vi "RT_main.vi"() -> ()   [LabVIEW 2013]
uses:
  <vilib>/NI/STM/compatibility/stm_MetaDataElement.ctl
  <vilib>/Platform/TimedLoop/XDataNode/timing_clust.ctl
  <vilib>/Platform/TimedLoop/XDataNode/nitl_modes.ctl
  <vilib>/Platform/TimedLoop/XDataNode/wakeup.ctl
  <vilib>/NI/STM/compatibility/stm_TCP Read Options.ctl
  <vilib>/rvi/interface/common/niFpgaWaitOnOcc.vi
  <vilib>/NI/STM/TCP/Get Connection Reference (TCP).vi
  <vilib>/NI/STM/TCP/Write Meta Data (TCP Ref).vi
  <vilib>/FPGAPlugInAG/cRIO-9101/niLvFpga_Open_cRIO-9101.vi
  <vilib>/rvi/interface/common/dynamic/niFpgaDynamicAddResources.vi
  <vilib>/FPGAPlugInAG/Dynamic/niLvFpga_Reset_Dynamic.vi
  <vilib>/FPGAPlugInAG/Dynamic/niLvFpga_Run_Dynamic.vi
  <vilib>/Utility/error.llb/Error Cluster From Error Code.vi
  <vilib>/rvi/errors/niLvFpgaAdjustHostInterfaceError.vi
  <vilib>/NI/STM/TCP/Read Message (TCP).vi
  <vilib>/NI/STM/TCP/Write Message (TCP).vi
  <vilib>/FPGAPlugInAG/Dynamic/niLvFpga_Close_Dynamic.vi
  <vilib>/Platform/TimedLoop/XDataNode/XDataNode.xnode
  <vilib>/rvi/interface/nirviOpenFPGA/nirviOpenFPGA.xnode
  FPGA Bitfiles/ForceClamp_FPGATarget_FPGAMain_Jp-CpyR53JY.lvbitx
  FPGA_Main.vi
  <vilib>/rvi/interface/nirviMethod/nirviMethod.xnode
  <vilib>/rvi/interface/nirviReadWriteControl/nirviReadWriteControl.xnode
  <vilib>/rvi/interface/nirviCloseFPGA/nirviCloseFPGA.xnode
  <vilib>/rvi/errors/niLvFpgaMergeErrorWithErrorCode.vi
  <vilib>/NI/STM/NI STM.lvlib
  <vilib>/rvi/interface/Simulation/niFpgaSimulationCallBeginRW.vi
  <vilib>/FPGAPlugInAG/Dynamic/niLvFpga_StartFifo_Dynamic.vi
  <vilib>/FPGAPlugInAG/Dynamic/niLvFpga_ReadFifo_Dynamic.vi
  <vilib>/FPGAPlugInAG/Dynamic/niLvFpga_ConfigureFifo_Dynamic.vi
  <vilib>/Platform/TimedLoop/XDataNode/XDNodeRunTimeDep.lvlib
  <vilib>/FPGAPlugInAG/Dynamic/niLvFpga_StopFifo_Dynamic.vi
  <vilib>/FPGAPlugInAG/Dynamic/niLvFpga_WriteFifo_Dynamic.vi
  NiFpgaLv.dll
panel:
  out "Receive Loop Timing":u32
  out "New waveTable":bool
  in  "Repeat mode":bool
  out "Data":fxp<+/-,20,5>[](array[numeric])
  out "Send Loop Timing":u32
  out "Connection OK":bool
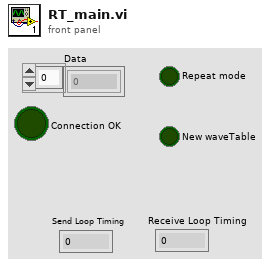
[diagram p1: front panel]
types:
  T1 = typedef "stm_MetaDataElement.ctl" = string
  T2 = typedef "Semaphore RefNum" = refnum<k1>
  T3 = typedef "NI STM.lvlib/TCP Connection Info.ctl" = cluster{"connection ID":refnum<k5>, "Meta data":T4[]}
  T4 = typedef "NI STM.lvlib/MetaDataElement.ctl" = string
  T5 = typedef "XDNodeRunTimeDep.lvlib/timing_clust.ctl" = cluster{"Expected End [f-1]":u64, "Actual End [f-1]":u64, "Finished Late? [f-1]":bool, "Expected End [i-1]":u64, "Actual End [i-1]":u64, "Finished Late? [i-1]":bool, "Expected Start [i]":u64, "Actual Start [i]":u64, "Expected Start [f]":u64, "Actual Start [f]":u64, "Source Name":string, "Structure Name":string, "Period":i64, "Deadline":i64, "Offset":i64, "Start":i64, "Priority":i32, "Timeout":i32, "Mode":T6, "Wakeup Reason":T7, "Error":errorcluster, "Source Type":string, "Secondary Source Type":string, "Global End Time":u64, "Global Start Time":u64, "Frame Duration":u64, "Iteration Duration":u64, "Assigned CPU":i32, "I/O Scan Engine Mode":u32}
  T6 = typedef "XDNodeRunTimeDep.lvlib/nitl_modes.ctl" = enum32{"No Change", "Process missed periods, maintain original phase", "Discard missed periods, maintain original phase", "Process missed periods, ignore original phase", "Discard missed periods, ignore original phase"}
  T7 = typedef "XDNodeRunTimeDep.lvlib/wakeup.ctl" = enum32{"Normal", "Aborted", "Asynchronous wakeup", "Timing source error", "Timed loop error", "Timeout"}
  T8 = typedef "stm_TCP Read Options.ctl" = cluster{"Ignore Timeout Error":bool, "timeout ms (1000)":i32}
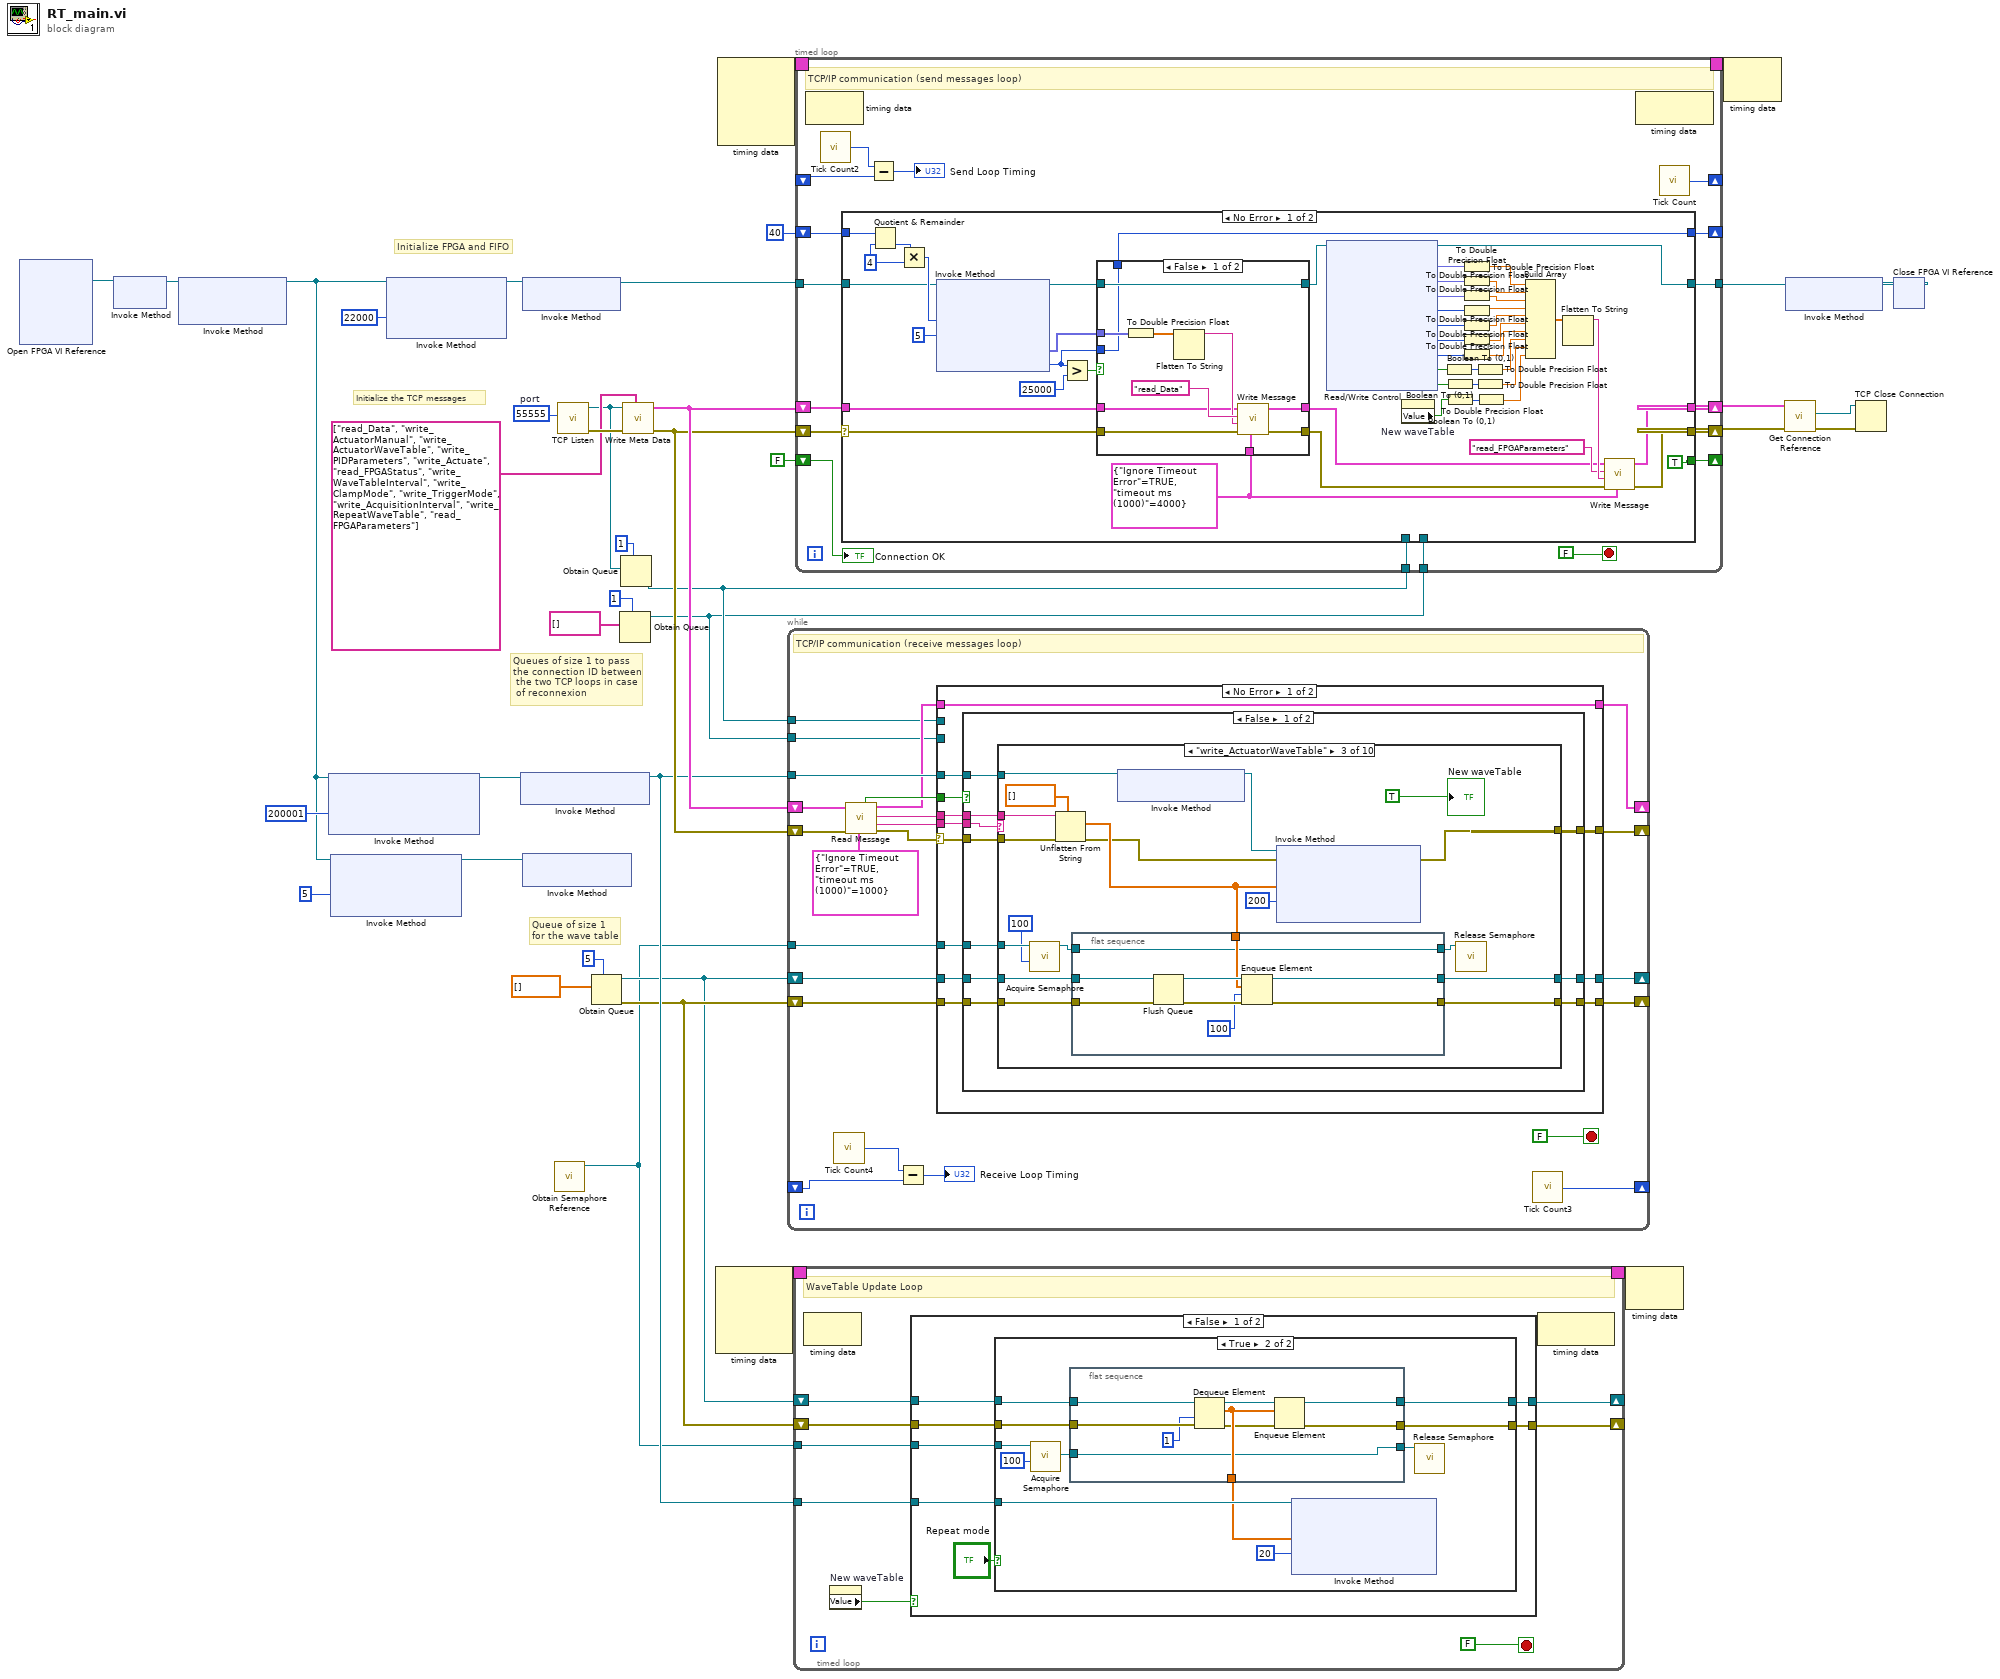
[diagram p0: block diagram]
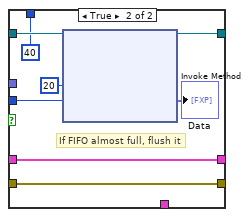
[diagram p2: hidden frame]
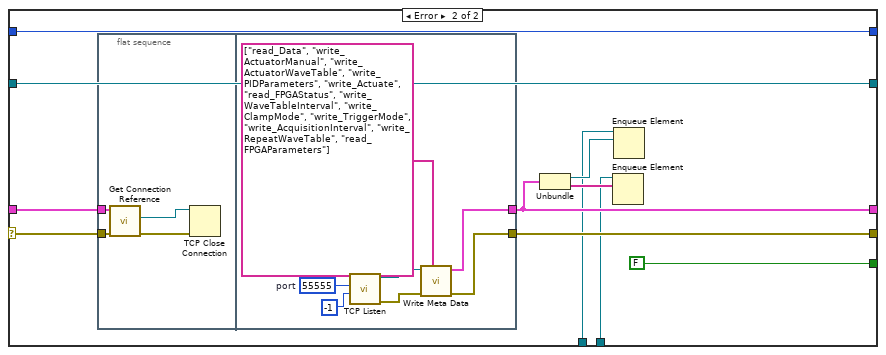
[diagram p3: hidden frame]
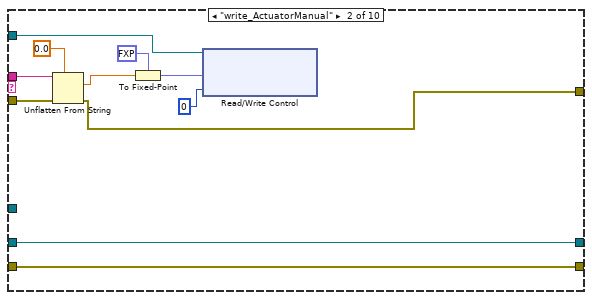
[diagram p5: hidden frame]
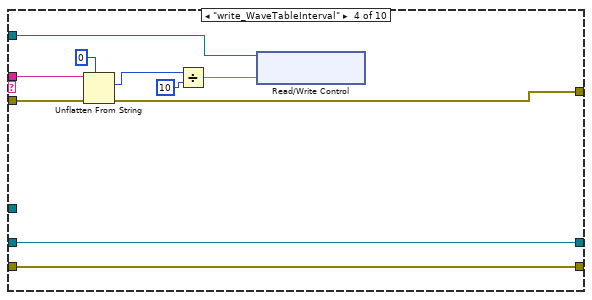
[diagram p6: hidden frame]
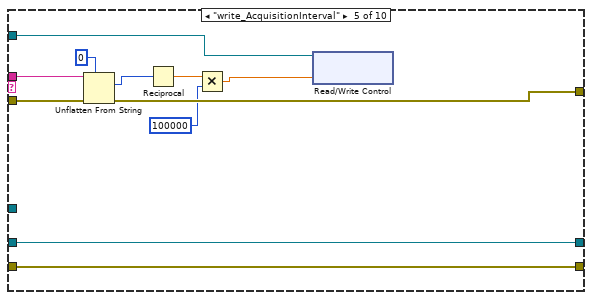
[diagram p7: hidden frame]
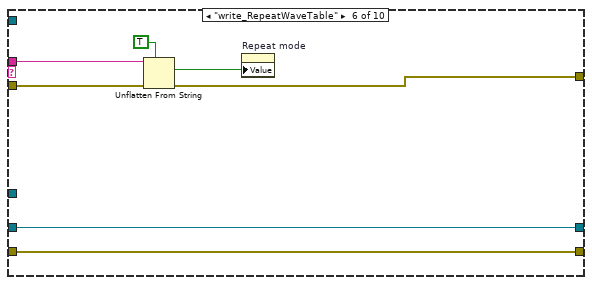
[diagram p8: hidden frame]
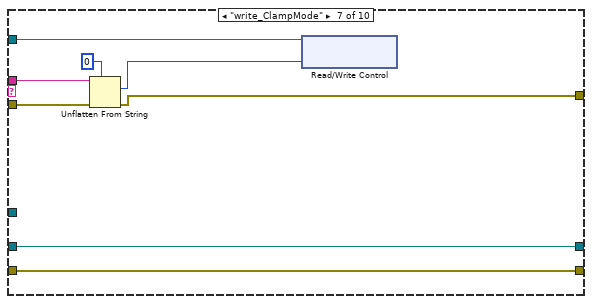
[diagram p9: hidden frame]
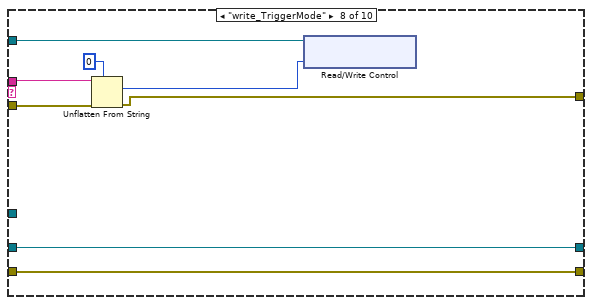
[diagram p10: hidden frame]
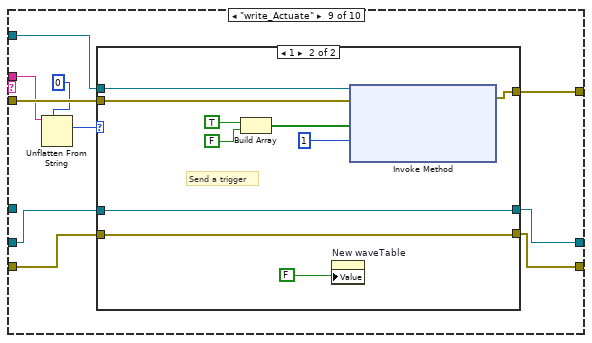
[diagram p11: hidden frame]
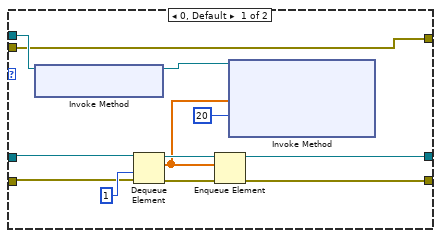
[diagram p12: hidden frame]
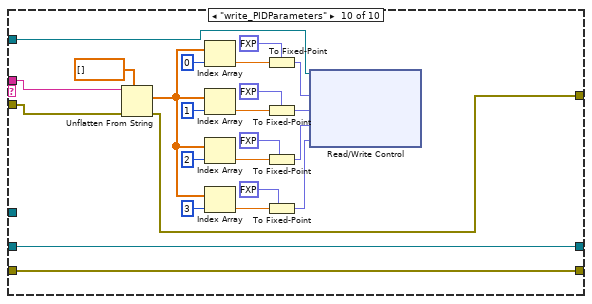
[diagram p13: hidden frame]
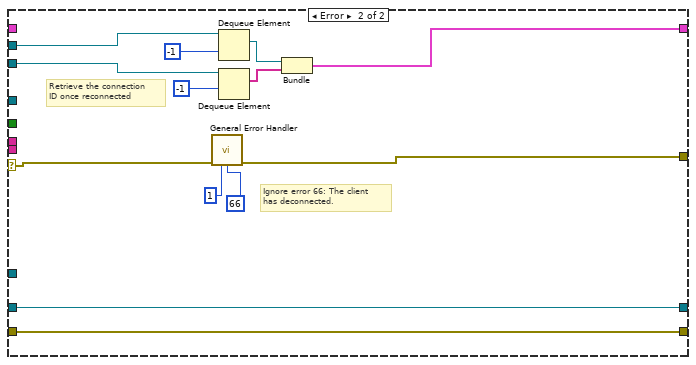
[diagram p15: hidden frame]
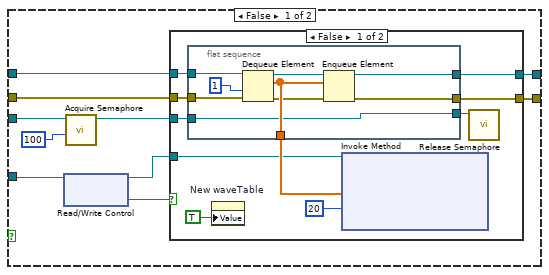
[diagram p16: hidden frame]
diagram:
  w34 = u16 55555  # port
  # "Queue of size 1 \nfor the wave table"
  # "Queues of size 1 to pass\nthe connection ID between\n the two TCP loops in case\n of reconnexion"
  # "Initialize the TCP messages"
  # "Initialize FPGA and FIFO"
  n1 = xnode "Open FPGA VI Reference"() -> ("FPGA VI Reference Out"=w1:refnum<k20>)  [unwired: 2 in, 1 out]
  n2 = xnode "Invoke Method"("FPGA VI Reference In"=w1) -> ("FPGA VI Reference Out"=w7:refnum<k20>)  [unwired: 1 in, 1 out]
  n3 = xnode "Invoke Method"("FPGA VI Reference In"=w7) -> ("FPGA VI Reference Out"=w6:refnum<k20>)  [unwired: 2 in, 1 out]
  n4 = xnode "Invoke Method"("FPGA VI Reference In"=w6, "Requested Depth"=200001) -> ("FPGA VI Reference Out"=w17:refnum<k20>)  [unwired: 1 in, 2 out]
  n5 = xnode "Invoke Method"("FPGA VI Reference In"=w6, "Requested Depth"=5) -> ("FPGA VI Reference Out"=w14:refnum<k20>)  [unwired: 1 in, 2 out]
  n6 = xnode "Invoke Method"("FPGA VI Reference In"=w6, "Requested Depth"=22000) -> ("FPGA VI Reference Out"=w39:refnum<k20>)  [unwired: 1 in, 2 out]
  n7 = xnode "Invoke Method"("FPGA VI Reference In"=w17) -> ("FPGA VI Reference Out"=w10:refnum<k20>)  [unwired: 1 in, 1 out]
  n8 = xnode "Invoke Method"("FPGA VI Reference In"=w39) -> ("FPGA VI Reference Out"=w5:refnum<k20>)  [unwired: 1 in, 1 out]
  n9 = xnode "Invoke Method"("FPGA VI Reference In"=w14) -> ()  [unwired: 1 in, 2 out]
  n10 = call <vilib>:"Obtain Semaphore Reference.vi"() -> ("semaphore"=w2:T2)  [unwired: 5 in, 2 out]
  n11 = call <vilib>:"TCP Listen.vi"("port"=w34) -> ("error out"=w33:errorcluster, "connection ID"=w23:refnum<k5>)  [unwired: 3 in, 6 out]
  n12 = Obtain Queue(max queue size (-1, unlimited)=5, element data type=dbl[] []) -> (queue out=w8:refnum<queue>, error out=w9:errorcluster)  [unwired: 3 in, 1 out]
  n13 = Obtain Queue(max queue size (-1, unlimited)=1, element data type=string[] []) -> (queue out=w21:refnum<queue>)  [unwired: 3 in, 2 out]
  n14 = Obtain Queue(max queue size (-1, unlimited)=1, element data type=w23) -> (queue out=w22:refnum<queue>)  [unwired: 3 in, 2 out]
  n15 = call-poly <vilib>:"Write Meta Data.vi"("Meta data"=T1[] ["read_Data", "write_ActuatorManual", "write_ActuatorWaveTable", "write_PIDParameters", "write_Actuate", "read_FPGAStatus", "write_WaveTableInterval", "write_ClampMode", "write_TriggerMode", "write_AcquisitionInterval", "write_RepeatWaveTable", "read_FPGAParameters"], "error in"=w33, "connection ID"=w23) -> ("error out"=w27:errorcluster, "Connection Info Out"=w28:T3)  [unwired: 7 in]
  n16 = node-c288() -> (w12:T5)  [unwired: 4 in]
  n17 = node-c288() -> (w4:T5)  [unwired: 4 in]
  n18 = while "RT OS->Host Message Parser" {
    shift-right: [w51] -> _
    shift-left: w28 -> [w61]
    shift-right: [w53] -> _
    shift-left: w27 -> [w60]
    tunnel: w10 -> [w54]
    tunnel: w22 -> [w50]
    tunnel: w21 -> [w49]
    shift-right: [w47] -> _
    shift-left: w8 -> [w45]
    shift-right: [w48] -> _
    shift-left: w9 -> [w46]
    shift-right: [w43] -> _
    shift-left: _ -> [w42]
    tunnel: w2 -> [w40]
    stop <- FALSE stop-if-true
    # "TCP/IP communication (receive messages loop)"
    n19 = call "Tick Count4"() -> ("Tick Count(mSec)"=w41:u32)
    n20 = call-poly <vilib>:"Read Message.vi"("Options"=T8 {"Ignore Timeout Error"=TRUE, "timeout ms (1000)"=1000}, "error in"=w60, "Connection Info"=w61) -> ("error out"=w57:errorcluster, "Name"=w59:T4, "data string"=w58:string, "Connection Info Out"=w52:T3, "Timed Out?"=w56:bool)  [unwired: 3 in, 1 out]
    n21 = Subtract(x=w41, y=w42) -> (x-y=→"Receive Loop Timing":u32)
    n22 = case shown="No Error" w57 {
      selector: w57 -> [w71 w234]
      tunnel: w59 -> [w74 _]
      tunnel: w58 -> [w73 _]
      tunnel: w56 -> [w72 _]
      tunnel: [w70 w233] -> w53
      tunnel: w54 -> [w69 _]
      tunnel: [w68 w237] -> w51
      tunnel: w52 -> [w68 _]
      tunnel: w50 -> [_ w241]
      tunnel: w49 -> [_ w240]
      tunnel: w45 -> [w67 w230]
      tunnel: w46 -> [w66 w229]
      tunnel: [w65 w230] -> w47
      tunnel: [w64 w229] -> w48
      tunnel: w40 -> [w63 _]
      frame No Error {
        n23 = case shown="False" w72 {
          tunnel: w74 -> [w81 _]
          tunnel: w73 -> [w84 _]
          tunnel: w71 -> [w83 w228]
          tunnel: [w82 w228] -> w70
          tunnel: w69 -> [w80 _]
          tunnel: w67 -> [w79 w227]
          tunnel: w66 -> [w78 w226]
          tunnel: [w77 w227] -> w65
          tunnel: [w76 w226] -> w64
          tunnel: w63 -> [w75 _]
          frame False {
            n24 = case shown="\"write_ActuatorWaveTable\"" w81 {
              tunnel: w84 -> [_ w98 w116 w132 w143 w152 w157 w167 w176 w224]
              tunnel: w83 -> [w87 w97 w115 w133 w144 w151 w156 w165 w178 w223]
              tunnel: [w87 w95 w99 w131 w142 w149 w155 w164 w177 w202] -> w82
              tunnel: w80 -> [_ w92 w107 w129 w140 _ w158 w166 w179 w225]
              tunnel: w79 -> [w86 w90 w113 w135 w146 w148 w161 w163 w173 w222]
              tunnel: w78 -> [w85 w89 w112 w134 w145 w147 w160 w162 w172 w221]
              tunnel: [w86 w90 w111 w135 w146 w148 w161 w163 w171 w222] -> w77
              tunnel: [w85 w89 w110 w134 w145 w147 w160 w162 w170 w221] -> w76
              tunnel: w75 -> [_ _ w104 _ _ _ _ _ _ _]
              frame Default {
              }
              frame "write_ActuatorManual" {
                n25 = Unflatten From String(type=0.0, binary string=w98, error in (no error)=w97) -> (value=w93:dbl, error out=w95:errorcluster)  [unwired: 3 out]
                n26 = To Fixed-Point(fixed-point type=fxp<+/-,20,5> 0.0, number=w93) -> (fixed-point=w91:fxp<+/-,20,5>)
                n27 = xnode "Read/Write Control"("FPGA VI Reference In"=w92, "tag_ManualSetPoint"=w91, "tag_ActuationMode"=0) -> ()  [unwired: 1 in, 2 out]
              }
              frame "write_ActuatorWaveTable" {
                n28 = call <vilib>:"Acquire Semaphore.vi"("ms timeout (-1)"=100, "semaphore"=w104) -> ("semaphore out"=w102:T2)  [unwired: 3 in, 2 out]
                n29 = Unflatten From String(type=dbl[] [], binary string=w116, error in (no error)=w115) -> (value=w108:dbl[], error out=w100:errorcluster)  [unwired: 3 out]
                n30 = flat-sequence {
                  tunnel: w113 -> [w125]
                  tunnel: w112 -> [w124]
                  tunnel: [w122] -> w111
                  tunnel: [w121] -> w110
                  tunnel: w108 -> [w118]
                  tunnel: [w117] -> w103
                  tunnel: w102 -> [w117]
                  frame #0 {
                    n31 = Flush Queue(queue=w125, error in (no error)=w124) -> (queue out=w120:refnum<queue>, error out=w123:errorcluster)  [unwired: 1 out]
                    n32 = Enqueue Element(queue=w120, element=w118, timeout in ms (-1)=100, error in (no error)=w123) -> (queue out=w122:refnum<queue>, error out=w121:errorcluster)  [unwired: 1 out]
                  }
                }
                n33 = xnode "Invoke Method"("FPGA VI Reference In"=w107) -> ("FPGA VI Reference Out"=w106:refnum<k20>)  [unwired: 1 in, 1 out]
                n34 = xnode "Invoke Method"("FPGA VI Reference In"=w106, "error in"=w100, "Data"=w108, "Timeout (ms)"=200) -> ("error out"=w99:errorcluster)  [unwired: 2 out]
                n35 = call <vilib>:"Release Semaphore.vi"("semaphore"=w103) -> ()  [unwired: 5 in, 2 out]
                "New waveTable" <- TRUE
              }
              frame "write_WaveTableInterval" {
                n36 = Unflatten From String(type=0, binary string=w132, error in (no error)=w133) -> (value=w126:i32, error out=w131:errorcluster)  [unwired: 3 out]
                n37 = Divide(x=w126, y=10) -> (x/y=w128:dbl)
                n38 = xnode "Read/Write Control"("FPGA VI Reference In"=w129, "tag_ActuationFreq"=w128) -> ()  [unwired: 1 in, 2 out]
              }
              frame "write_AcquisitionInterval" {
                n39 = Unflatten From String(type=0, binary string=w143, error in (no error)=w144) -> (value=w139:i32, error out=w142:errorcluster)  [unwired: 3 out]
                n40 = Reciprocal(x=w139) -> (1/x=w138:dbl)
                n41 = Multiply(x=w138, y=100000) -> (x*y=w136:dbl)
                n42 = xnode "Read/Write Control"("FPGA VI Reference In"=w140, "tag_AcqFreq"=w136) -> ()  [unwired: 1 in, 2 out]
              }
              frame "write_RepeatWaveTable" {
                n43 = Unflatten From String(type=TRUE, binary string=w152, error in (no error)=w151) -> (value=w150:bool, error out=w149:errorcluster)  [unwired: 3 out]
                n44 = property on="Repeat mode" class="Bool (strict)"("Value"=w150) -> ()  [unwired: 2 in, 2 out]
              }
              frame "write_ClampMode" {
                n45 = Unflatten From String(type=0, binary string=w157, error in (no error)=w156) -> (value=w154:i32, error out=w155:errorcluster)  [unwired: 3 out]
                n46 = xnode "Read/Write Control"("FPGA VI Reference In"=w158, "tag_ClampMode"=w154) -> ()  [unwired: 1 in, 2 out]
              }
              frame "write_TriggerMode" {
                n47 = Unflatten From String(type=0, binary string=w167, error in (no error)=w165) -> (value=w168:i32, error out=w164:errorcluster)  [unwired: 3 out]
                n48 = xnode "Read/Write Control"("FPGA VI Reference In"=w166, "tag_ActuationMode"=w168) -> ()  [unwired: 1 in, 2 out]
              }
              frame "write_Actuate" {
                n49 = Unflatten From String(type=0, binary string=w176) -> (value=w174:i32)  [unwired: 1 in, 4 out]
                n50 = case shown="1" w174 {
                  tunnel: w179 -> [w191 w199]
                  tunnel: w178 -> [w190 w198]
                  tunnel: [w190 w197] -> w177
                  tunnel: w173 -> [w184 w201]
                  tunnel: w172 -> [w183 w200]
                  tunnel: [w182 w201] -> w171
                  tunnel: [w181 w200] -> w170
                  frame 0, Default {
                    n51 = xnode "Invoke Method"("FPGA VI Reference In"=w191) -> ("FPGA VI Reference Out"=w180:refnum<k20>)  [unwired: 1 in, 1 out]
                    n52 = Dequeue Element(queue=w184, timeout in ms (-1)=1, error in (no error)=w183) -> (queue out=w188:refnum<queue>, element=w187:dbl[], error out=w186:errorcluster)  [unwired: 1 out]
                    n53 = Enqueue Element(queue=w188, element=w187, error in (no error)=w186) -> (queue out=w182:refnum<queue>, error out=w181:errorcluster)  [unwired: 1 in, 1 out]
                    n54 = xnode "Invoke Method"("FPGA VI Reference In"=w180, "Data"=w187, "Timeout (ms)"=20) -> ()  [unwired: 1 in, 3 out]
                  }
                  frame 1 {
                    # "Send a trigger"
                    n55 = Build Array(TRUE, FALSE) -> (w194:bool[])
                    n56 = property on="New waveTable" class="Bool (strict)"("Value"=FALSE) -> ()  [unwired: 2 in, 2 out]
                    n57 = xnode "Invoke Method"("FPGA VI Reference In"=w199, "error in"=w198, "Data"=w194, "Timeout (ms)"=1) -> ("error out"=w197:errorcluster)  [unwired: 2 out]
                  }
                }
              }
              frame "write_PIDParameters" {
                n58 = Unflatten From String(type=dbl[] [], binary string=w224, error in (no error)=w223) -> (value=w205:dbl[], error out=w202:errorcluster)  [unwired: 3 out]
                n59 = Index Array(array=w205, index=0) -> (element=w218:dbl)
                n60 = Index Array(array=w205, index=1) -> (element=w213:dbl)
                n61 = Index Array(array=w205, index=2) -> (element=w210:dbl)
                n62 = Index Array(array=w205, index=3) -> (element=w206:dbl)
                n63 = To Fixed-Point(fixed-point type=fxp<+,24,8> 0.0, number=w218) -> (fixed-point=w217:fxp<+,24,8>)
                n64 = To Fixed-Point(fixed-point type=fxp<+,24,8> 0.0, number=w213) -> (fixed-point=w212:fxp<+,24,8>)
                n65 = To Fixed-Point(fixed-point type=fxp<+,32,8> 0.0, number=w210) -> (fixed-point=w204:fxp<+,32,8>)
                n66 = To Fixed-Point(fixed-point type=fxp<+,20,4> 0.0, number=w206) -> (fixed-point=w203:fxp<+,20,4>)
                n67 = xnode "Read/Write Control"("FPGA VI Reference In"=w225, "Pgain"=w217, "Igain"=w212, "Dgain"=w204, "AntiWindupInterval"=w203) -> ()  [unwired: 1 in, 2 out]
              }
            }
          }
          frame True {
          }
        }
      }
      frame Error {
        # "Ignore error 66: The client\nhas deconnected."
        # "Retrieve the connection\nID once reconnected"
        n68 = call <vilib>:"General Error Handler.vi"("error in (no error)"=w234, "[exception action] (none:0)"=1, "[exception code]"=66) -> ("error out"=w233:errorcluster)  [unwired: 8 in, 4 out]
        n69 = Dequeue Element(queue=w241, timeout in ms (-1)=-1) -> (element=w239:refnum<k5>)  [unwired: 1 in, 3 out]
        n70 = Dequeue Element(queue=w240, timeout in ms (-1)=-1) -> (element=w238:string[])  [unwired: 1 in, 3 out]
        n71 = Bundle("connection ID"=w239, w238) -> (w237:cluster{"connection ID":refnum<k5>, string[]})  [unwired: 1 in]
      }
    }
    n72 = call "Tick Count3"() -> ("Tick Count(mSec)"=w43:u32)
  }
  n73 = timed-loop {
    timing: w12 -> [_]
    timing-out: [_] -> w11
    tunnel: w10 -> [w247]
    shift-right: [w246] -> _
    shift-left: w8 -> [w248]
    shift-right: [w245] -> _
    shift-left: w9 -> [w249]
    tunnel: w2 -> [w244]
    stop <- FALSE stop-if-true
    # "WaveTable Update Loop"
    n74 = node-c288() -> ()  [unwired: 1 in, 1 out]
    n75 = property on="New waveTable" class="Bool (strict)"() -> ("Value"=w243:bool)  [unwired: 2 in, 2 out]
    n76 = case shown="False" w243 {
      tunnel: w249 -> [w256 w308]
      tunnel: w248 -> [w255 w309]
      tunnel: w247 -> [w254 _]
      tunnel: [w252 w309] -> w246
      tunnel: [w251 w308] -> w245
      tunnel: w244 -> [w250 _]
      frame False {
        n77 = case shown="True" "Repeat mode" {
          tunnel: w254 -> [w262 w298]
          tunnel: w256 -> [w263 w296]
          tunnel: w255 -> [w264 w297]
          tunnel: [w266 w293] -> w252
          tunnel: [w265 w292] -> w251
          tunnel: w250 -> [w259 w291]
          frame False {
            n78 = xnode "Read/Write Control"("FPGA VI Reference In"=w262) -> ("FPGA VI Reference Out"=w261:refnum<k20>, "Actuating"=w260:bool)  [unwired: 1 in, 1 out]
            n79 = call <vilib>:"Acquire Semaphore.vi"("ms timeout (-1)"=100, "semaphore"=w259) -> ("semaphore out"=w258:T2)  [unwired: 3 in, 2 out]
            n80 = case shown="False" w260 {
              tunnel: [w274 w287] -> w266
              tunnel: [w273 w286] -> w265
              tunnel: w264 -> [w272 w287]
              tunnel: w263 -> [w271 w286]
              tunnel: w261 -> [w270 _]
              tunnel: w258 -> [w268 _]
              frame False {
                n81 = flat-sequence {
                  tunnel: [w283] -> w276
                  tunnel: [w281] -> w274
                  tunnel: [w280] -> w273
                  tunnel: w272 -> [w279]
                  tunnel: w271 -> [w278]
                  tunnel: [w277] -> w269
                  tunnel: w268 -> [w277]
                  frame #0 {
                    n82 = Dequeue Element(queue=w279, timeout in ms (-1)=1, error in (no error)=w278) -> (queue out=w284:refnum<queue>, element=w283:dbl[], error out=w282:errorcluster)  [unwired: 1 out]
                    n83 = Enqueue Element(queue=w284, element=w283, error in (no error)=w282) -> (queue out=w281:refnum<queue>, error out=w280:errorcluster)  [unwired: 1 in, 1 out]
                  }
                }
                n84 = property on="New waveTable" class="Bool (strict)"("Value"=TRUE) -> ()  [unwired: 2 in, 2 out]
                n85 = xnode "Invoke Method"("FPGA VI Reference In"=w270, "Data"=w276, "Timeout (ms)"=20) -> ()  [unwired: 1 in, 3 out]
                n86 = call <vilib>:"Release Semaphore.vi"("semaphore"=w269) -> ()  [unwired: 5 in, 2 out]
              }
              frame True {
              }
            }
          }
          frame True {
            n87 = call <vilib>:"Acquire Semaphore.vi"("ms timeout (-1)"=100, "semaphore"=w291) -> ("semaphore out"=w289:T2)  [unwired: 3 in, 2 out]
            n88 = flat-sequence {
              tunnel: w297 -> [w307]
              tunnel: w296 -> [w306]
              tunnel: [w303] -> w295
              tunnel: [w301] -> w293
              tunnel: [w300] -> w292
              tunnel: [w299] -> w290
              tunnel: w289 -> [w299]
              frame #0 {
                n89 = Dequeue Element(queue=w307, timeout in ms (-1)=1, error in (no error)=w306) -> (queue out=w304:refnum<queue>, element=w303:dbl[], error out=w302:errorcluster)  [unwired: 1 out]
                n90 = Enqueue Element(queue=w304, element=w303, error in (no error)=w302) -> (queue out=w301:refnum<queue>, error out=w300:errorcluster)  [unwired: 1 in, 1 out]
              }
            }
            n91 = xnode "Invoke Method"("FPGA VI Reference In"=w298, "Data"=w295, "Timeout (ms)"=20) -> ()  [unwired: 1 in, 3 out]
            n92 = call <vilib>:"Release Semaphore.vi"("semaphore"=w290) -> ()  [unwired: 5 in, 2 out]
          }
        }
      }
      frame True {
      }
    }
    n93 = node-c288() -> ()  [unwired: 1 in, 1 out]
  }
  n94 = timed-loop {
    shift-right: [w328] -> _
    shift-left: FALSE -> [w325]
    shift-right: [w326] -> w29
    shift-left: w27 -> [w322]
    shift-right: [w327] -> w30
    shift-left: w28 -> [w323]
    tunnel: w21 -> [w321]
    tunnel: w22 -> [w320]
    tunnel: w5 -> [w319]
    tunnel: [w318] -> w19
    shift-right: [w316] -> _
    shift-left: u32 40 -> [w317]
    shift-right: [w314] -> _
    shift-left: _ -> [w313]
    timing: w4 -> [_]
    timing-out: [_] -> w3
    stop <- FALSE stop-if-true
    # "TCP/IP communication (send messages loop)"
    n95 = node-c288() -> ()  [unwired: 1 in, 1 out]
    n96 = call "Tick Count2"() -> ("Tick Count(mSec)"=w312:u32)
    n97 = case shown="No Error" w322 {
      selector: w322 -> [w376 w407]
      tunnel: w323 -> [w377 w408]
      tunnel: [w353 w406] -> w326
      tunnel: [w354 w405] -> w327
      tunnel: [TRUE FALSE] -> w328
      tunnel: w321 -> [_ w402]
      tunnel: w320 -> [_ w401]
      tunnel: w319 -> [w364 w400]
      tunnel: [w363 w400] -> w318
      tunnel: w317 -> [w373 w399]
      tunnel: [w365 w399] -> w316
      frame No Error {
        w343 = T8 {"Ignore Timeout Error"=TRUE, "timeout ms (1000)"=4000} ("Options")
        w374 = u32 4
        n98 = Quotient & Remainder(x=w373, y=w374) -> (floor(x/y)=w375:u32)  [unwired: 1 out]
        n99 = Multiply(x=w375, y=w374) -> (x*y=w367:u32)
        n100 = xnode "Invoke Method"("FPGA VI Reference In"=w364, "Number of Elements"=w367, "Timeout (ms)"=5) -> ("FPGA VI Reference Out"=w369:refnum<k20>, "Data"=w368:fxp<+/-,20,5>[], "Elements Remaining"=w366:u32)  [unwired: 1 in, 1 out]
        n101 = Greater?(x=w366, y=u32 25000) -> (0:w370:bool)
        n102 = case shown="False" w370 {
          tunnel: w369 -> [w383 w397]
          tunnel: [w383 w396] -> w342
          tunnel: w368 -> [w382 _]
          tunnel: w377 -> [w387 w395]
          tunnel: w376 -> [w386 w394]
          tunnel: [w385 w395] -> w331
          tunnel: [w384 w394] -> w332
          tunnel: w366 -> [w381 w392]
          tunnel: [w381 u32 40] -> w365
          tunnel: w343 -> [w380 _]
          frame False {
            n103 = To Double Precision Float(number=w382) -> (double precision float=w379:dbl[])
            n104 = Flatten To String(anything=w379) -> (data string=w388:string)  [unwired: 3 in, 2 out]
            n105 = call-poly <vilib>:"Write Message.vi"("Options"=w380, "error in (no error)"=w386, "Data"=w388, "Name"="read_Data", "Connection Info"=w387) -> ("error out"=w384:errorcluster, "Connection Info Out"=w385:T3)  [unwired: 5 in]
          }
          frame True {
            # "If FIFO almost full, flush it"
            n106 = xnode "Invoke Method"("FPGA VI Reference In"=w397, "Number of Elements"=w392, "Timeout (ms)"=20) -> ("FPGA VI Reference Out"=w396:refnum<k20>, "Data"=→"Data":fxp<+/-,20,5>[])  [unwired: 1 in, 2 out]
          }
        }
        n107 = xnode "Read/Write Control"("FPGA VI Reference In"=w342) -> ("FPGA VI Reference Out"=w363:refnum<k20>, "Pgain"=w351:fxp<+,24,8>, "Igain"=w350:fxp<+,24,12>, "Dgain"=w349:fxp<+,32,8>, "tag_ClampMode"=w348:i32, "tag_ActuationMode"=w347:i32, "tag_AcqFreq"=w346:i32, "tag_ActuationFreq"=w345:i32, "FIFO Full"=w338:bool, "Actuating"=w337:bool)  [unwired: 1 in, 1 out]
        n108 = property on="New waveTable" class="Bool (strict)"() -> ("Value"=w333:bool)  [unwired: 2 in, 2 out]
        n109 = Boolean To (0,1)(Boolean=w338) -> (0, 1=w340:i16)
        n110 = Boolean To (0,1)(Boolean=w337) -> (0, 1=w339:i16)
        n111 = Boolean To (0,1)(Boolean=w333) -> (0, 1=w344:i16)
        n112 = To Double Precision Float(number=w351) -> (double precision float=w362:dbl)
        n113 = To Double Precision Float(number=w350) -> (double precision float=w361:dbl)
        n114 = To Double Precision Float(number=w349) -> (double precision float=w360:dbl)
        n115 = To Double Precision Float(number=w348) -> (double precision float=w359:dbl)
        n116 = To Double Precision Float(number=w347) -> (double precision float=w358:dbl)
        n117 = To Double Precision Float(number=w346) -> (double precision float=w357:dbl)
        n118 = To Double Precision Float(number=w345) -> (double precision float=w356:dbl)
        n119 = To Double Precision Float(number=w340) -> (double precision float=w336:dbl)
        n120 = To Double Precision Float(number=w339) -> (double precision float=w335:dbl)
        n121 = To Double Precision Float(number=w344) -> (double precision float=w334:dbl)
        n122 = Build Array(w362, w361, w360, w359, w358, w357, w356, w336, w335, w334) -> (w341:dbl[])
        n123 = Flatten To String(anything=w341) -> (data string=w355:string)  [unwired: 3 in, 2 out]
        n124 = call-poly <vilib>:"Write Message.vi"("Options"=w343, "error in (no error)"=w332, "Data"=w355, "Name"="read_FPGAParameters", "Connection Info"=w331) -> ("error out"=w353:errorcluster, "Connection Info Out"=w354:T3)  [unwired: 5 in]
      }
      frame Error {
        n125 = flat-sequence {
          tunnel: w408 -> [w410]
          tunnel: w407 -> [w409]
          tunnel: [w415] -> w405
          tunnel: [w414] -> w406
          frame #0 {
            n126 = call-poly <vilib>:"Get Connection Reference.vi"("error in"=w409, "Connection Info"=w410) -> ("error out"=w411:errorcluster, "connection ID out"=w412:refnum<k5>)  [unwired: 7 in, 1 out]
            n127 = TCP Close Connection(connection ID=w412, error in (no error)=w411) -> ()  [unwired: 1 in, 2 out]
          }
          frame #1 {
            w419 = u16 55555  # port
            n128 = call <vilib>:"TCP Listen.vi"("timeout ms (wait forever: -1)"=-1, "port"=w419) -> ("error out"=w417:errorcluster, "connection ID"=w418:refnum<k5>)  [unwired: 2 in, 6 out]
            n129 = call-poly <vilib>:"Write Meta Data.vi"("Meta data"=T1[] ["read_Data", "write_ActuatorManual", "write_ActuatorWaveTable", "write_PIDParameters", "write_Actuate", "read_FPGAStatus", "write_WaveTableInterval", "write_ClampMode", "write_TriggerMode", "write_AcquisitionInterval", "write_RepeatWaveTable", "read_FPGAParameters"], "error in"=w417, "connection ID"=w418) -> ("error out"=w414:errorcluster, "Connection Info Out"=w415:T3)  [unwired: 7 in]
          }
        }
        n130 = Unbundle(w405) -> ("connection ID"=w403:refnum<k5>, "Meta data"=w404:T4[])
        n131 = Enqueue Element(queue=w402, element=w404) -> ()  [unwired: 2 in, 3 out]
        n132 = Enqueue Element(queue=w401, element=w403) -> ()  [unwired: 2 in, 3 out]
      }
    }
    n133 = Subtract(x=w312, y=w313) -> (x-y=→"Send Loop Timing":u32)
    n134 = node-c288() -> ()  [unwired: 1 in, 1 out]
    n135 = call "Tick Count"() -> ("Tick Count(mSec)"=w314:u32)
    "Connection OK" <- w325
  }
  n136 = node-c288(w11) -> ()  [unwired: 1 out]
  n137 = node-c288(w3) -> ()  [unwired: 1 out]
  n138 = call-poly <vilib>:"Get Connection Reference.vi"("error in"=w29, "Connection Info"=w30) -> ("error out"=w35:errorcluster, "connection ID out"=w36:refnum<k5>)  [unwired: 7 in, 1 out]
  n139 = xnode "Invoke Method"("FPGA VI Reference In"=w19) -> ("FPGA VI Reference Out"=w37:refnum<k20>)  [unwired: 1 in, 1 out]
  n140 = TCP Close Connection(connection ID=w36, error in (no error)=w35) -> ()  [unwired: 1 in, 2 out]
  n141 = xnode "Close FPGA VI Reference"("FPGA VI Reference In"=w37) -> ()  [unwired: 1 in, 1 out]
